vi "ThisIsATestIII.vi"() -> ()   [LabVIEW 2016]
panel:
  in  "Break line":bool
  out "continuous?":bool
  out "ready to fire":bool
  in  "Arm Flag":bool
  in  "stop":bool
  out "timer":dbl
  out "wait timer":dbl
  out "Loop":dbl
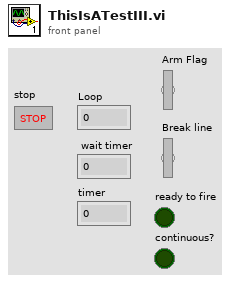
[diagram p1: front panel]
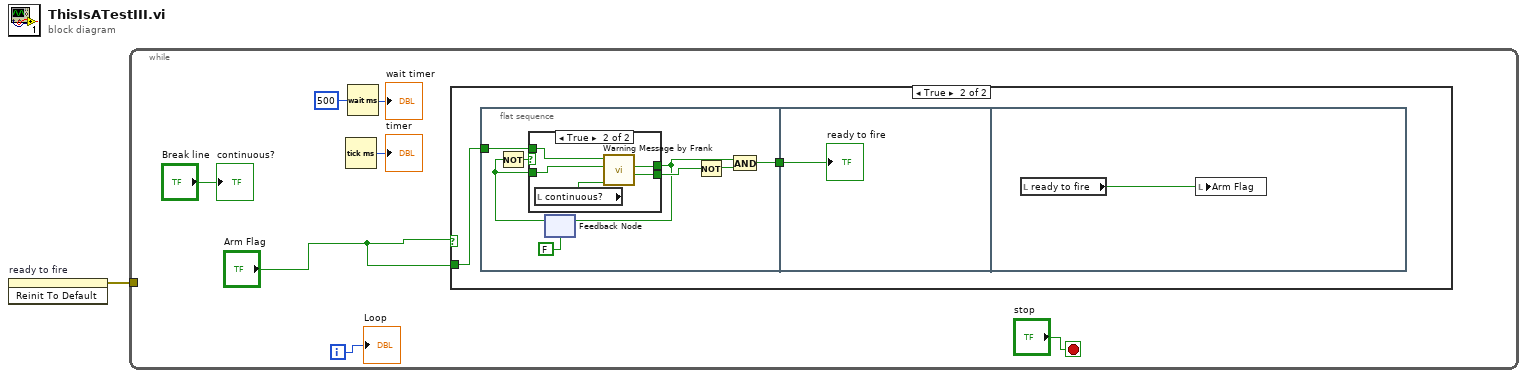
[diagram p0: block diagram]
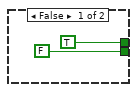
[diagram p3: hidden frame]
diagram:
  n1 = invoke on="ready to fire" class="Bool (strict)" method="Reinit To Default"() -> (error out=w1:errorcluster)  [unwired: 3 in, 2 out]
  n2 = while {
    tunnel: w1 -> [_]
    i -> [w8]
    stop <- "stop" stop-if-true
    n3 = Tick Count (ms)() -> (millisecond timer value=→"timer":u32)
    n4 = Wait (ms)(milliseconds to wait=u32 500) -> (millisecond timer value=→"wait timer":u32)
    n5 = case shown="True" "Arm Flag" {
      tunnel: "Arm Flag" -> [_ w9]
      frame False {
      }
      frame True {
        n6 = flat-sequence {
          tunnel: w9 -> [w15]
          tunnel: [w17] -> w10
          tunnel: w10 -> [w26]
          frame #0 {
            n7 = feedback #1(FALSE) -> (w11:bool)
            n8 = Not(x=w11) -> (.not. x?=w12:bool)
            n9 = case shown="True" w12 {
              tunnel: [TRUE w23] -> w13
              tunnel: [FALSE w25] -> w16
              tunnel: w15 -> [_ w24]
              tunnel: w11 -> [_ w22]
              frame False {
              }
              frame True {
                n10 = local read "continuous?"() -> (w21:bool)
                n11 = call "Warning Message by Frank.vi"("Contiuous"=w21, "ok?"=w22, "Arm Flag"=w24) -> ("super cancel"=w25:bool, "super ok"=w23:bool)  [unwired: 6 in, 1 out]
              }
            }
            n12 = feedback-in #1(w13) -> ()
            n13 = Not(x=w16) -> (.not. x?=w18:bool)
            n14 = And(x=w13, y=w18) -> (x .and. y?=w17:bool)
          }
          frame #1 {
            "ready to fire" <- w26
          }
          frame #2 {
            n15 = local read "ready to fire"() -> (w27:bool)
            n16 = local write "Arm Flag"(w27) -> ()
          }
        }
      }
    }
    "Loop" <- w8
    "continuous?" <- "Break line"
  }
